vi "DataPacker_LogReconnectionAttempt.vi"(8 "error in (no error)":errorcluster, 11 "DataPacker in":refnum<class "DataPacker.lvclass">) -> (0 "error out":errorcluster, 3 "DataPacker out":refnum<class "DataPacker.lvclass">)   [LabVIEW 2018, in "feGEM DataPacker.lvlib" / "DataPacker.lvclass"]
uses:
  DataPacker.lvclass
  DataPacker.lvclass/DataPacker.ctl
  <vilib>/Utility/SystemLogging/NI_SystemLogging.lvlib
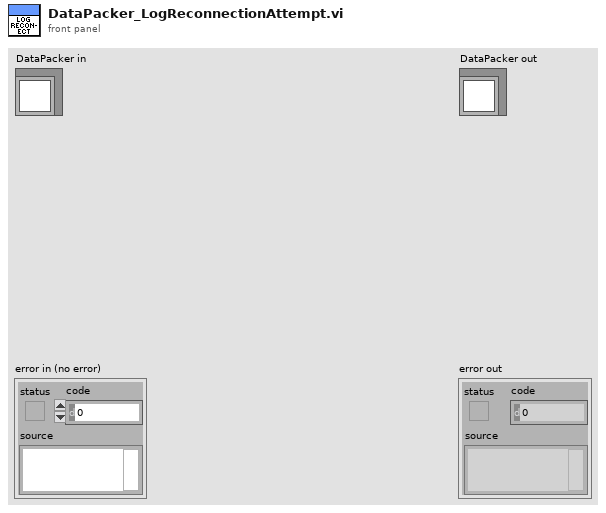
[diagram p1: front panel]
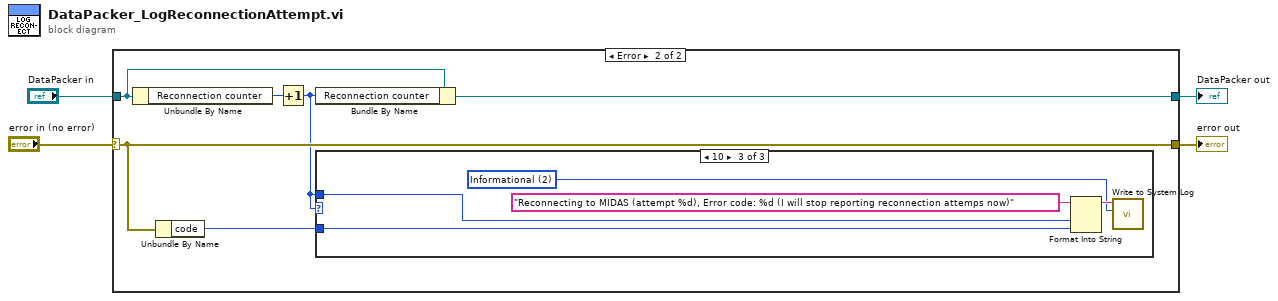
[diagram p0: block diagram]
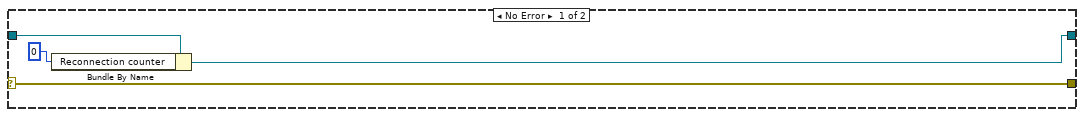
[diagram p2: hidden frame]
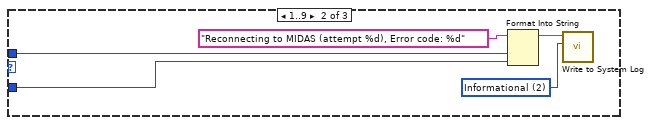
[diagram p4: hidden frame]
diagram:
  n1 = case shown="Error" "error in (no error)" {
    selector: "error in (no error)" -> [w8 w13]
    tunnel: [w8 w13] -> w3
    tunnel: [w6 w14] -> w1
    tunnel: "DataPacker in" -> [w7 w12]
    frame No Error {
      n2 = Bundle By Name(cluster=w7, "Reconnection counter"=0) -> (w6:refnum<class "DataPacker.lvclass">)
    }
    frame Error {
      n3 = Unbundle By Name(w12) -> ("Reconnection counter"=w11:i32)
      n4 = Unbundle By Name(w13) -> ("code"=w9:i32)
      n5 = Increment(x=w11) -> (x+1=w10:i32)
      n6 = Bundle By Name(cluster=w12, "Reconnection counter"=w10) -> (w14:refnum<class "DataPacker.lvclass">)
      n7 = case shown="10" w10 {
        tunnel: w10 -> [_ w17 w22]
        tunnel: w9 -> [_ w16 w21]
        frame 0, Default {
        }
        frame 1..9 {
          w15 = 2 items=["Error", "Warning", "Informational"] ("severity")
          n8 = Format Into String(initial string="Reconnecting to MIDAS (attempt %d), Error code: %d" ("message"), w17, w16) -> (resulting string=w19:string)  [unwired: 2 in, 1 out]
          n9 = call <vilib>:"Write to System Log.vi"("severity"=w15, "message"=w19) -> ()  [unwired: 9 in, 1 out]
        }
        frame 10 {
          w20 = 2 items=["Error", "Warning", "Informational"] ("severity")
          n10 = Format Into String(initial string="Reconnecting to MIDAS (attempt %d), Error code: %d (I will stop reporting reconnection attemps now)" ("message"), w22, w21) -> (resulting string=w24:string)  [unwired: 2 in, 1 out]
          n11 = call <vilib>:"Write to System Log.vi"("severity"=w20, "message"=w24) -> ()  [unwired: 9 in, 1 out]
        }
      }
    }
  }
  "error out" <- w3
  "DataPacker out" <- w1
